vi "FTW-Project-DiscoverBuildSpecs.vi"(0 "Project Ref (blank for Active Project)":refnum<vi>, 5 "Filter by Type (blank for all)":string, 11 "error in":errorcluster) -> (4 "Project Ref out":refnum<vi>, 6 "Build Spec ItemIDs":string[](array[string]), 8 "Build Spec Display Names":string[](array[string]), 10 "Build Spec Display Types":string[](array[string]), 15 "error out":errorcluster)   [LabVIEW 2012]
uses:
  Core/Error/FTW-ERR-ThrowError.vi
panel:
  # "Inputs"
  # "Outputs"
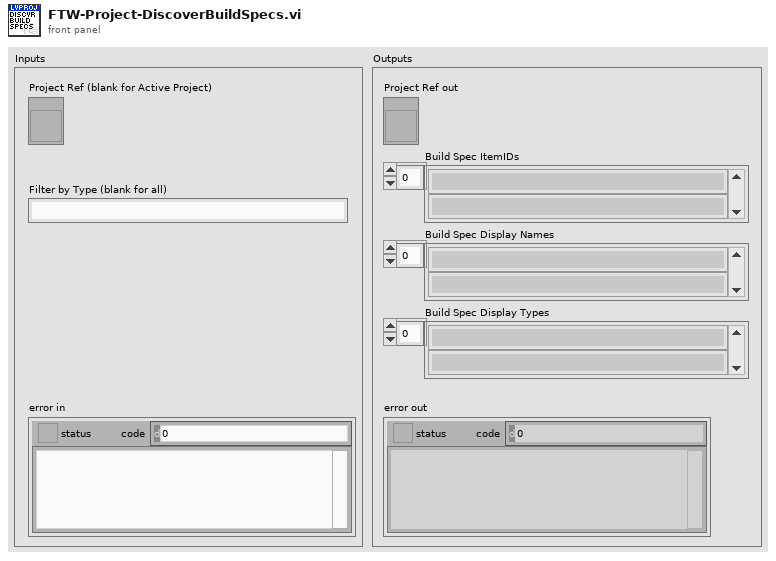
[diagram p1: front panel]
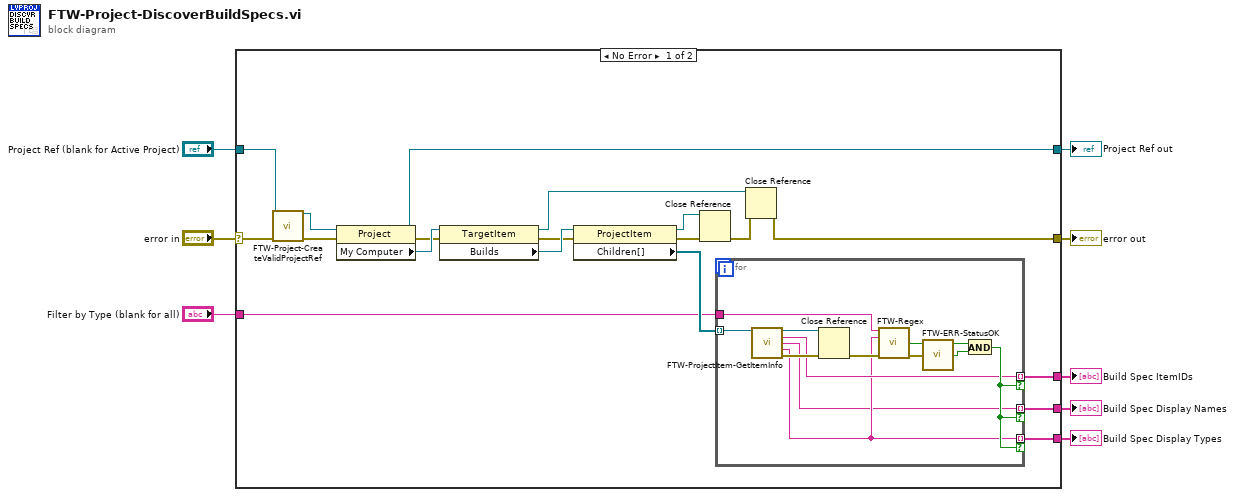
[diagram p0: block diagram]
diagram:
  n1 = case shown="No Error" "error in" {
    selector: "error in" -> [w10 w41]
    tunnel: [w14 w41] -> w8
    tunnel: [w22 _] -> w2
    tunnel: [w21 _] -> w1
    tunnel: "Project Ref (blank for Active Project)" -> [w9 w40]
    tunnel: "Filter by Type (blank for all)" -> [w20 _]
    tunnel: [w19 _] -> w3
    tunnel: [w13 w40] -> w4
    frame No Error {
      n2 = call "FTW-Project-CreateValidProjectRef.vi"("Project Ref (blank for Active Project)"=w9, "error in"=w10) -> ("Project Ref"=w12:refnum<vi>, "error out"=w11:errorcluster)  [unwired: 11 in, 1 out]
      n3 = property class="Project"(reference=w12, error in=w11) -> (reference out=w13:refnum<vi>, error out=w24:errorcluster, "My Computer"=w27:refnum<vi>)
      n4 = property class="TargetItem"(reference=w27, error in=w24) -> (reference out=w18:refnum<vi>, error out=w23:errorcluster, "Builds"=w26:refnum<vi>)
      n5 = property class="ProjectItem"(reference=w26, error in=w23) -> (reference out=w17:refnum<vi>, error out=w16:errorcluster, "Children[]"=w25:refnum<vi>[])
      n6 = Close Reference(reference=w17, error in (no error)=w16) -> (error out=w15:errorcluster)
      n7 = for {
        tunnel: w25 -> [w36] mode=indexing
        tunnel: [w30] -> w22 mode=indexing if=w39
        tunnel: [w32] -> w21 mode=indexing if=w39
        tunnel: w20 -> [w38]
        tunnel: [w31] -> w19 mode=indexing if=w39
        n8 = call "FTW-ProjectItem-GetItemInfo.vi"("ProjectItem"=w36) -> ("ProjectItem out"=w35:refnum<vi>, "ItemID"=w32:string, "Display Name"=w30:string, "Item Type GUID"=w31:string, "error out"=w34:errorcluster)  [unwired: 10 in]
        n9 = Close Reference(reference=w35, error in (no error)=w34) -> (error out=w33:errorcluster)
        n10 = call "FTW-Regex.vi"("Regular Expression"=w38, "Input String"=w31, "error in"=w33) -> ("Match Found?"=w37:bool, "error out"=w29:errorcluster)  [unwired: 8 in, 3 out]
        n11 = call "FTW-ERR-StatusOK.vi"("error to check"=w29) -> ("Status OK?"=w28:bool)
        n12 = And(x=w37, y=w28) -> (x .and. y?=w39:bool)
      }
      n13 = Close Reference(reference=w18, error in (no error)=w15) -> (error out=w14:errorcluster)
    }
    frame Error {
    }
  }
  "error out" <- w8
  "Build Spec Display Types" <- w3
  "Build Spec Display Names" <- w2
  "Build Spec ItemIDs" <- w1
  "Project Ref out" <- w4
